vi "RemoveArgumentAndComments.vi"(7 "AllCaseStates":string[](array[string]), 11 "TransactionStateIn":string) -> (1 "Comment":string, 2 "Argument":string, 3 "TransactionStateOut":string)   [LabVIEW 2012, in "StateReverse.lvclass"]
uses:
  <resource>/Framework/Providers/Open_GDS/UML/StateReverse_class/StateReverse.lvclass
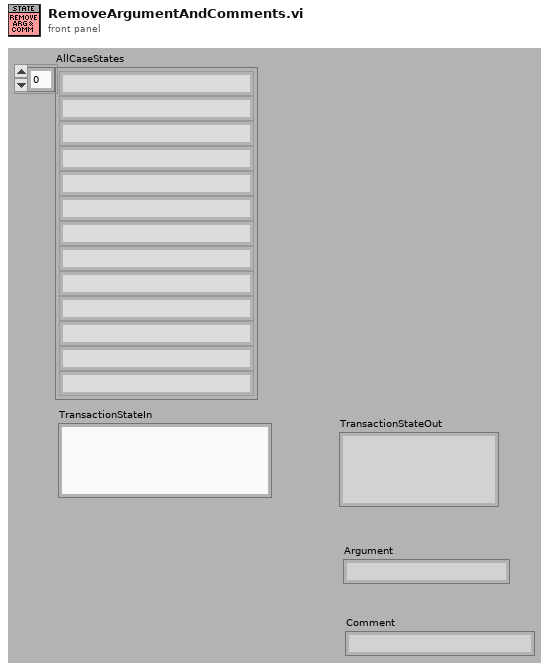
[diagram p1: front panel]
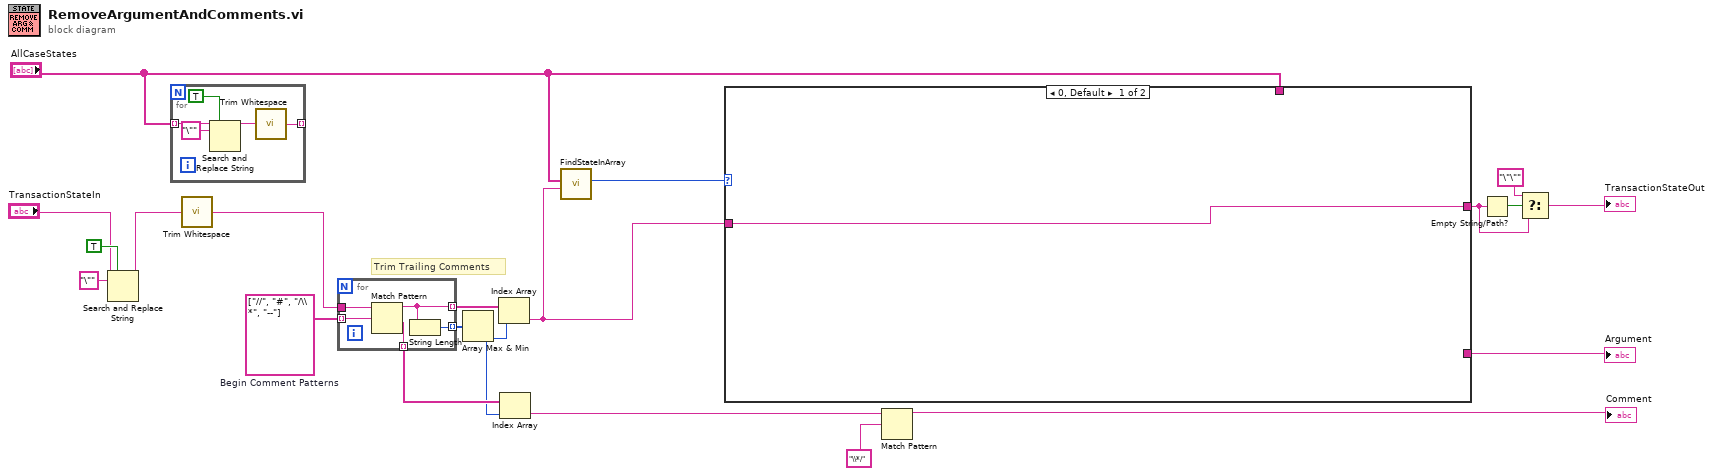
[diagram p0: block diagram]
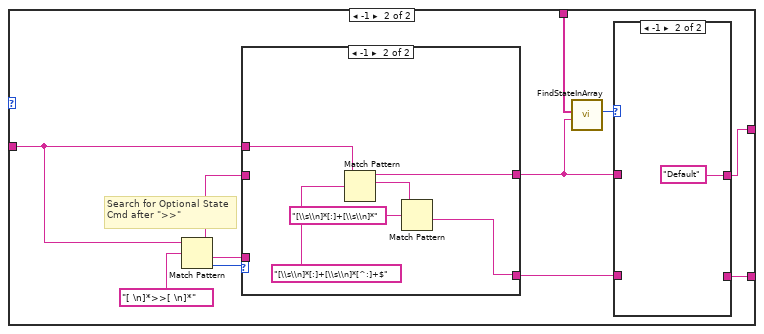
[diagram p2: hidden frame]
diagram:
  w21 = string[] ["//", "#", "/\\*", "--"]  # Begin Comment Patterns
  # "Trim Trailing Comments"
  n1 = Search and Replace String(replace all?=TRUE ("replace all? (F)"), input string="TransactionStateIn", search string="\"") -> (result string=w8:string)  [unwired: 5 in, 3 out]
  n2 = for {
    tunnel: "AllCaseStates" -> [w24] mode=indexing
    tunnel: [w22] -> _ mode=indexing
    n3 = Search and Replace String(replace all?=TRUE ("replace all? (F)"), input string=w24, search string="\"") -> (result string=w23:string)  [unwired: 5 in, 3 out]
    n4 = call <vilib>:"Trim Whitespace.vi"("string"=w23) -> ("trimmed string"=w22:string)  [unwired: 1 in]
  }
  n5 = call <vilib>:"Trim Whitespace.vi"("string"=w8) -> ("trimmed string"=w12:string)  [unwired: 1 in]
  n6 = for {
    tunnel: w12 -> [w31]
    tunnel: [w29] -> w19 mode=indexing
    tunnel: w21 -> [w30] mode=indexing
    tunnel: [w28] -> w20 mode=indexing
    tunnel: [w27] -> w17 mode=indexing
    n7 = Match Pattern(string=w31, regular expression=w30) -> (before substring=w29:string, after substring=w27:string)  [unwired: 1 in, 2 out]
    n8 = String Length(string=w29) -> (length=w28:i32)
  }
  n9 = Array Max & Min(array=w20) -> (min index (indices)=w16:i32)  [unwired: 3 out]
  n10 = Index Array(array=w19, index=w16) -> (element=w7:string)
  n11 = Index Array(array=w17, index=w16) -> (element=w15:string)
  n12 = call <resource>:"FindStateInArray.vi"("TransactionState"=w7, "AllCaseStates"="AllCaseStates") -> ("index of element"=w2:i32)  [unwired: 7 in, 2 out]
  n13 = case shown="0, Default" w2 {
    tunnel: [w32 w37] -> w3
    tunnel: [_ w35] -> w18
    tunnel: "AllCaseStates" -> [_ w34]
    tunnel: w7 -> [w32 w33]
    frame 0, Default {
    }
    frame -1 {
      # "Search for Optional State Cmd after \">>\""
      n14 = Match Pattern(string=w33, regular expression="[ \n]*>>[ \n]*") -> (before substring=w41:string, after substring=w40:string, offset past match=w42:i32)  [unwired: 1 in, 1 out]
      n15 = case shown="-1" w42 {
        tunnel: w41 -> [w47 _]
        tunnel: [w47 w53] -> w38
        tunnel: [w48 w50] -> w36
        tunnel: w40 -> [w48 _]
        tunnel: w33 -> [_ w49]
        frame 0, Default {
        }
        frame -1 {
          n16 = Match Pattern(string=w49, regular expression="[\\s\\n]*[:]+[\\s\\n]*[^:]+$") -> (before substring=w53:string, match substring=w52:string)  [unwired: 1 in, 2 out]
          n17 = Match Pattern(string=w52, regular expression="[\\s\\n]*[:]+[\\s\\n]*") -> (after substring=w50:string)  [unwired: 1 in, 3 out]
        }
      }
      n18 = call <resource>:"FindStateInArray.vi"("TransactionState"=w38, "AllCaseStates"=w34) -> ("index of element"=w39:i32)  [unwired: 7 in, 2 out]
      n19 = case shown="-1" w39 {
        tunnel: w38 -> [w45 _]
        tunnel: [w45 "Default" ("TransactionStateIn")] -> w37
        tunnel: w36 -> [w44 _]
        tunnel: [w44 _] -> w35
        frame 0, Default {
        }
        frame -1 {
        }
      }
    }
  }
  "Argument" <- w18
  n20 = Match Pattern(string=w15, regular expression="\\*/") -> (before substring=→"Comment":string)  [unwired: 1 in, 3 out]
  n21 = Empty String/Path?(string/path=w3) -> (empty?=w5:bool)
  n22 = Select(t="\"\"" ("format string"), s=w5, f=w3) -> (s? t:f=→"TransactionStateOut":string)
